vi "Config VI.vi"(8 "error in (no error)":errorcluster, 11 "Plugin in":refnum<class "Plugin.lvclass">) -> (0 "error out":errorcluster, 3 "Plugin out":refnum<class "Plugin.lvclass">)   [LabVIEW 2015, in "HtmlReportPlugin.lvclass"]
uses:
  HtmlReportPlugin.lvclass
  Core/Plugin.lvclass
  Core/Plugin/Plugin Config UI State.ctl
  JsonReportPlugin.lvclass
panel:
  in  "Report Folder":string
  in  "Enable":bool
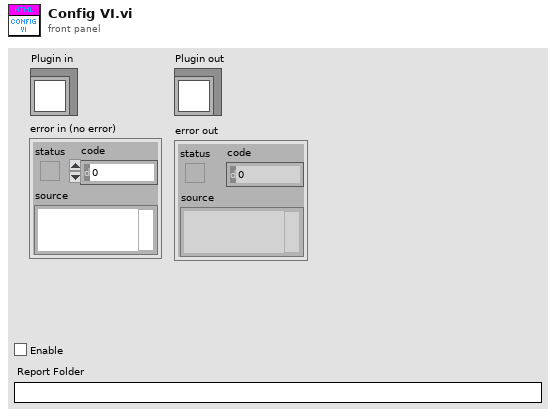
[diagram p1: front panel]
types:
  T1 = typedef "Plugin.lvclass/Plugin Config UI State.ctl" = enum16{"UI_LOOP", "INIT", "END"}
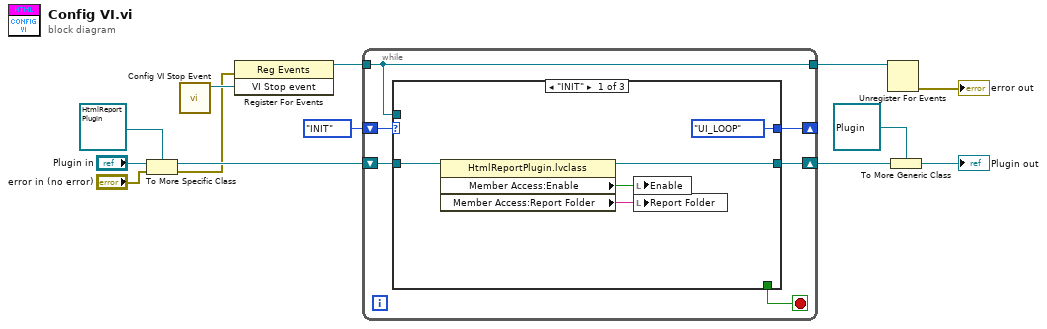
[diagram p0: block diagram]
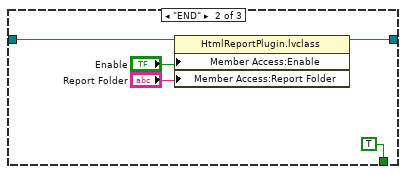
[diagram p2: hidden frame]
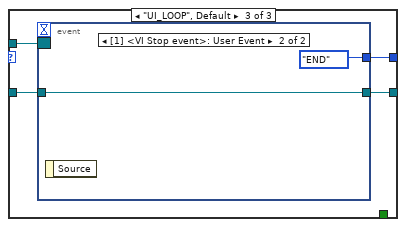
[diagram p3: hidden frame]
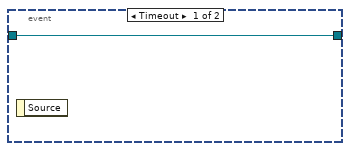
[diagram p4: hidden frame]
diagram:
  n1 = To More Specific Class(target class=refnum<class "HtmlReportPlugin.lvclass"> refnum ("HtmlReportPlugin.lvclass"), reference="Plugin in", error in="error in (no error)") -> (specific class reference=w9:refnum<class "HtmlReportPlugin.lvclass">, error out=w3:errorcluster)
  n2 = call "Config VI Stop Event.vi"() -> ("VI Stop event"=w13:refnum<user-event>)  [unwired: 11 in]
  n3 = register-events(error in=w3, w13) -> (reference out=w12:refnum<event-registration>)  [unwired: 1 in, 1 out]
  n4 = while {
    tunnel: w12 -> [w18]
    tunnel: [w18] -> w6
    shift-right: [w16] -> _
    shift-left: Plugin_Config_UI_State."INIT" ("State") -> [w17]
    shift-right: [w14] -> w8
    shift-left: w9 -> [w15]
    stop <- w19 stop-if-true
    n5 = case shown="\"INIT\"" w17 {
      tunnel: [_ TRUE _] -> w19
      tunnel: w18 -> [_ _ w33]
      tunnel: [Plugin_Config_UI_State."UI_LOOP" ("State") _ w32] -> w16
      tunnel: w15 -> [w23 w28 w31]
      tunnel: [w22 w27 w30] -> w14
      frame "INIT" {
        n6 = property class="HtmlReportPlugin.lvclass"(reference=w23) -> (reference out=w22:refnum<class "HtmlReportPlugin.lvclass">, "Member Access:Enable"=w21:bool, "Member Access:Report Folder"=w20:string)  [unwired: 1 in, 1 out]
        n7 = local write "Enable"(w21) -> ()
        n8 = local write "Report Folder"(w20) -> ()
      }
      frame "END" {
        n9 = property class="HtmlReportPlugin.lvclass"(reference=w28, "Member Access:Enable"="Enable", "Member Access:Report Folder"="Report Folder") -> (reference out=w27:refnum<class "HtmlReportPlugin.lvclass">)  [unwired: 1 in, 1 out]
      }
      frame "UI_LOOP", Default {
        n10 = event shown="[1] <VI Stop event>: User Event" {
          selector: w33 -> [_ _]
          dyn-events: _ -> [_ _]
          timeout: _ -> [_ _]
          tunnel: [_ Plugin_Config_UI_State."END" ("State")] -> w32
          tunnel: w31 -> [w34 w35]
          tunnel: [w34 w35] -> w30
          event Timeout {
            n11 = event-data() -> ()  [unwired: 1 in, 1 out]
          }
          event User Event {
            n12 = event-data() -> ()  [unwired: 1 in, 1 out]
          }
        }
      }
    }
  }
  n13 = Unregister For Events(event registration refnum=w6) -> (error out=→"error out":errorcluster)  [unwired: 1 in]
  n14 = To More Generic Class(target class=refnum<class "Plugin.lvclass"> refnum ("Plugin out"), reference=w8) -> (generic class reference=→"Plugin out":refnum<class "Plugin.lvclass">)
